vi "Teardown.vi"(7 "Actor in":refnum<class "Actor.lvclass">, 8 "Error in":errorcluster) -> (5 "Actor out":refnum<class "Actor.lvclass">)   [LabVIEW 2025, in "jettl.lvlib" / "Actor.lvlib"]
uses:
  Actor.lvlib
  Actor/Actor.lvclass
  Lifecycle.ctl
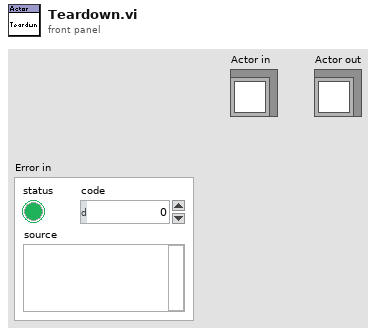
[diagram p1: front panel]
types:
  T1 = typedef "jettl.lvlib/Actor.lvlib/Lifecycle.ctl" = enum16{"Setup", "Teardown"}
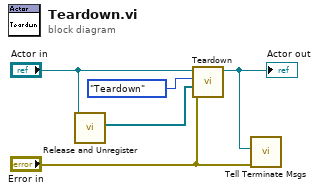
[diagram p0: block diagram]
diagram:
  n1 = call "Release and Unregister.vi"("Actor"="Actor in") -> ("Unhandled Msgs"=w4:refnum<class "Msg.lvclass">[])  [unwired: 10 in]
  n2 = call-dynamic "Teardown.vi"("Error in"="Error in", "Unhandled Msgs"=w4, "Lifecycle"=Lifecycle."Teardown", "Actor in"="Actor in") -> ("Actor out"=w2:refnum<class "Actor.lvclass">)  [unwired: 7 in]
  "Actor out" <- w2
  n3 = call "Tell Terminate Msgs.vi"("Error in"="Error in", "Actor"=w2) -> ()  [unwired: 10 in]
